vi "get Number Of Errors.vi"(8 "error in":errorcluster, 11 "cycloneHandle":u32) -> (0 "error out":errorcluster, 3 "function return":u32)   [LabVIEW 2021, in "CycloneControlSDK.lvlib"]
doc: "extern \"C\" uint32_t _cdecl getNumberOfErrors(uint32_t cycloneHandle);"
uses:
  CycloneControlSDK.lvlib
  CycloneControlSDK_64.dll
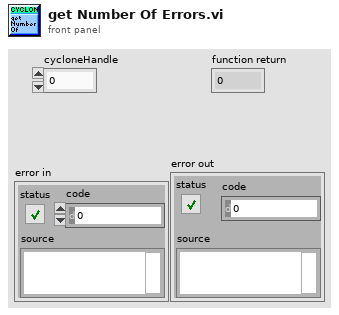
[diagram p1: front panel]
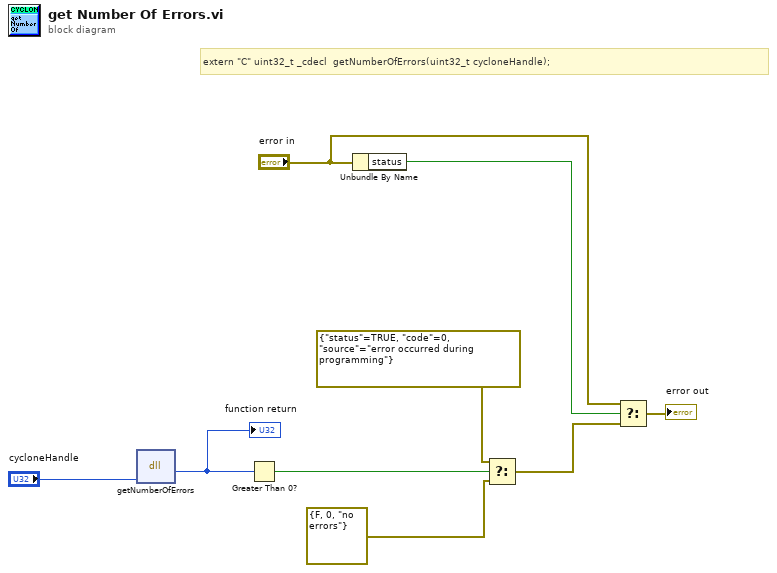
[diagram p0: block diagram]
diagram:
  # "extern \"C\" uint32_t _cdecl  getNumberOfErrors(uint32_t cycloneHandle);"
  n1 = dll-call lib="C:/PEMicro/cyclone/cycloneControl/controlsdk/examples/labview2018/user.lib/CycloneControlSDK/CycloneControlSDK_64.dll" fn="getNumberOfErrors"("cycloneHandle"="cycloneHandle") -> ("return type"=w8:u32)  [unwired: 4 in, 2 out]
  "function return" <- w8
  n2 = Greater Than 0?(x=w8) -> (x > 0?=w7:bool)
  n3 = Unbundle By Name("error in") -> ("status"=w4:bool)
  n4 = Select(t=errorcluster {"status"=TRUE, "code"=0, "source"="error occurred during programming"} ("error constant"), s=w7, f=errorcluster {"status"=FALSE, "code"=0, "source"="no errors"} ("error constant")) -> (s? t:f=w2:errorcluster)
  n5 = Select(t="error in", s=w4, f=w2) -> (s? t:f=→"error out":errorcluster)
